vi "服务端INI.vi"(0 "服务端配置":cluster{"本机 IP":string, "侦听端口":u16}={"本机 IP"="", "侦听端口"=4001}) -> (14 "侦听ID":refnum<k5>, 16 "可用？":bool)   [LabVIEW 2019, in "MainPage.lvlib" / "MainPage.lvclass"]
uses:
  MainPage.lvclass
panel:
  out "错误输出":errorcluster
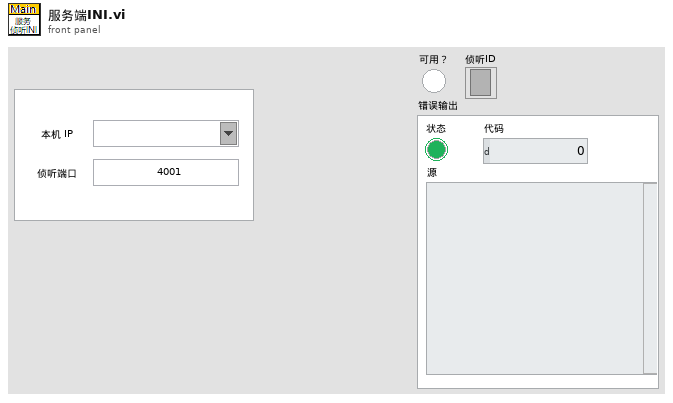
[diagram p1: front panel]
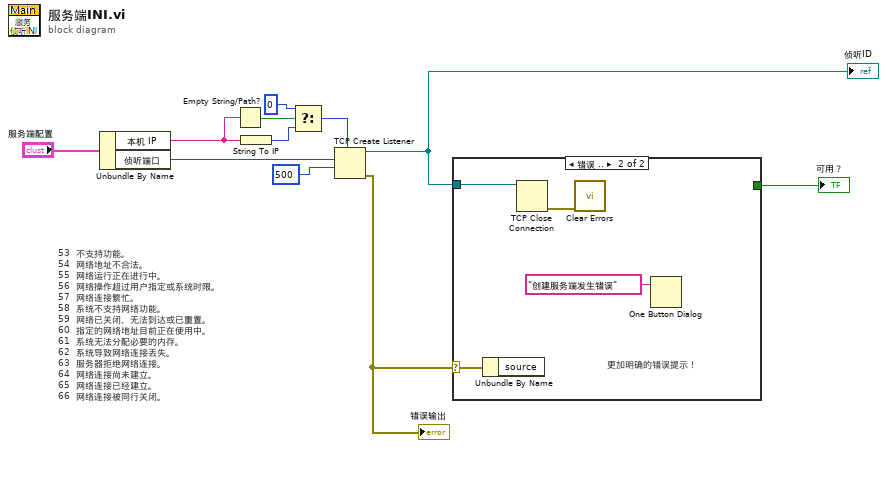
[diagram p0: block diagram]
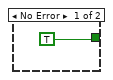
[diagram p2: hidden frame]
diagram:
  # "53  不支持功能。\n54  网络地址不合法。\n55  网络运行正在进行中。\n56  网络操作超过用户指定或系统时限。\n57  网络连接繁忙。\n58  系统不支持网络功能。\n59  网络已关闭、无法到达或已重置。\n60  指定的网络地址目前正在使用中。\n61  系统无法分配必要的内存。\n62  系统导致网络连接丢失。\n63  服务器拒绝网络连接。\n64  网络连接尚未建立。\n65  网络连接已经建立。\n66  网络连接被同行关闭。"
  n1 = Unbundle By Name("服务端配置") -> ("本机 IP"=w4:string, "侦听端口"=w5:u16)
  n2 = Empty String/Path?(string/path=w4) -> (empty?=w10:bool)
  n3 = String To IP(1:w4) -> (0:w9:u32)
  n4 = Select(t=u32 0, s=w10, f=w9) -> (s? t:f=w7:u32)
  n5 = TCP Create Listener(7:w7, 9:500 ("超时毫秒(25000)"), 10:w5) -> (0:w2:errorcluster, 3:w3:refnum<k5>)  [unwired: 2 in, 1 out]
  "侦听ID" <- w3
  "错误输出" <- w2
  n6 = case shown="错误 .." w2 {
    selector: w2 -> [_ w13]
    tunnel: w3 -> [_ w14]
    tunnel: [TRUE _] -> w1
    frame No Error {
    }
    frame Error {
      # "更加明确的错误提示！"
      n7 = Unbundle By Name(w13) -> ()  [unwired: 1 out]
      n8 = TCP Close Connection(connection ID=w14) -> (error out=w15:errorcluster)  [unwired: 2 in, 1 out]
      n9 = call <vilib>:"Clear Errors.vi"("error in (no error)"=w15) -> ()  [unwired: 5 in, 2 out]
      n10 = One Button Dialog(message="创建服务端发生错误" ("消息")) -> ()  [unwired: 1 in, 1 out]
    }
  }
  "可用？" <- w1
